vi "main_v6.vi"() -> ()   [LabVIEW 2024]
uses:
  <vilib>/Instr/_visa.llb/VISA Find Search Mode.ctl
  b10df30e-cdc0-40cb-bad4-31a4bb11d415.vi
  1b63e7fc-7b7c-41b1-b45b-52a754c22197.vi
  <vilib>/MakerHub/LINX/Public/Peripherals/Digital/Digital Write 1 Chan.vi
  <vilib>/MakerHub/LINX/Public/Peripherals/Digital/Digital Write N Chans.vi
  <vilib>/MakerHub/LINX/Private/Local IO/LinxDigitalWrite.vi
  <vilib>/MakerHub/LINX/Public/Utilities/Check Channel.vi
  <vilib>/MakerHub/LINX/Private/Local IO/Handle Errors.vi
  <vilib>/LabVIEW Open Source Project/MQTT TCP Connection/MQTT_TCP/Connection/TCPConnection.lvclass
  C:/Program Files (x86)/National Instruments/LabVIEW 2024/vi.lib/LabVIEW Open Source Project/Connection/Connection/Connection.lvclass
  <vilib>/LabVIEW Open Source Project/MQTT Client/Client class/Client.lvclass
  C:/Program Files (x86)/National Instruments/LabVIEW 2024/vi.lib/LabVIEW Open Source Project/MQTT Connection/MQTT_Base/Base Class/MQTT_Base.lvclass
  <vilib>/Instr/_visa.llb/VISA Configure Serial Port (Instr).vi
  <vilib>/MakerHub/LINX/Public/Utilities/Open Local.vi
  <vilib>/MakerHub/LINX/Private/Utilties/Generate Error.vi
  <vilib>/LabVIEW Open Source Project/MQTT Connection/MQTT_Base/Base Class/MQTT_Base.lvclass
  <vilib>/MakerHub/LINX/LMH-LINX.lvlib
panel:
  out "ambient temp":u8=6
  out "date":string
  out "is_heater_on":bool
  out "residents":u8=6
  out "activity state":i8
  out "Movement timer 2":u8
  out "door activity":bool
  out "Movement detected":bool
  out "Movement timer":u8
  out "Movement detected3":bool
  out "Is door open":bool
  out "Distance":dbl
  out "Pressure":u16
  out "Temperature":dbl
  in  "Pressure":u16
  in  "Distance":dbl
  in  "Temperature":dbl
  out "size(s)":i32
  out "unsigned byte array":u8[](array[numeric])
  out "after substring":string
  out "time string":string
  out "find list":string[](array[string])
  out "String":string
  in  "stop":bool
  in  "VISA Reciever":refnum<visa-resource-name>="ASRL1::INSTR"
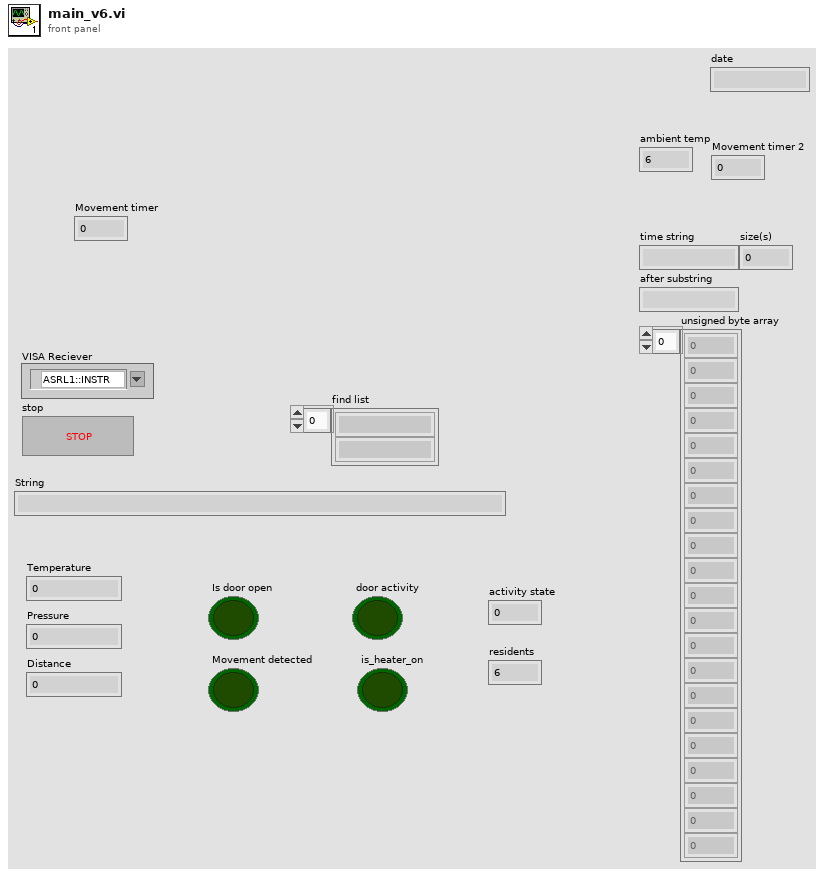
[diagram p1: front panel]
types:
  T1 = typedef "VISA Find Search Mode.ctl" = u32
  T2 = cluster{"is_door_open":bool, "is_heater_on":bool, "residents":u8, "temp":dbl, "pressure":u16, "timestamp":string, "date":string}
  T3 = typedef "LMH-LINX.lvlib/LINX Ref.ctl" = cluster{"IO":T4, "Interface":T5, "LINX Device Config":T6}
  T4 = typedef "LMH-LINX.lvlib/Platform.ctl" = enum16{"Remote", "Local"}
  T5 = typedef "LMH-LINX.lvlib/Interface.ctl" = enum16{"Serial", "TCP"}
  T6 = typedef "LMH-LINX.lvlib/Device.lvlib/LINX Device Config.ctl" = cluster{"Interface":T5, "COM Port":refnum<visa-resource-name>, "TCP Configuration":T7, "Device Family":u8, "Device ID":u8, "Device Name":string, "TCP Ref":refnum<k5>, "Channels":T8}
  T7 = typedef "LMH-LINX.lvlib/Device.lvlib/TCP Config.ctl" = cluster{"IP Address":string, "Port":u16}
  T8 = typedef "LMH-LINX.lvlib/Channels.ctl" = cluster{"DI":u8[], "DO":u8[], "AI":u8[], "AO":u8[], "PWM":u8[], "QE":u8[], "UART":u8[], "I2C 2":u8[], "SPI":u8[], "CAN":u8[], "Servo":u8[], "AI Ref (V)":dbl, "AI Resolution (Bits)":u8, "AO Ref (V)":dbl, "AO Resolution (Bits)":u8}
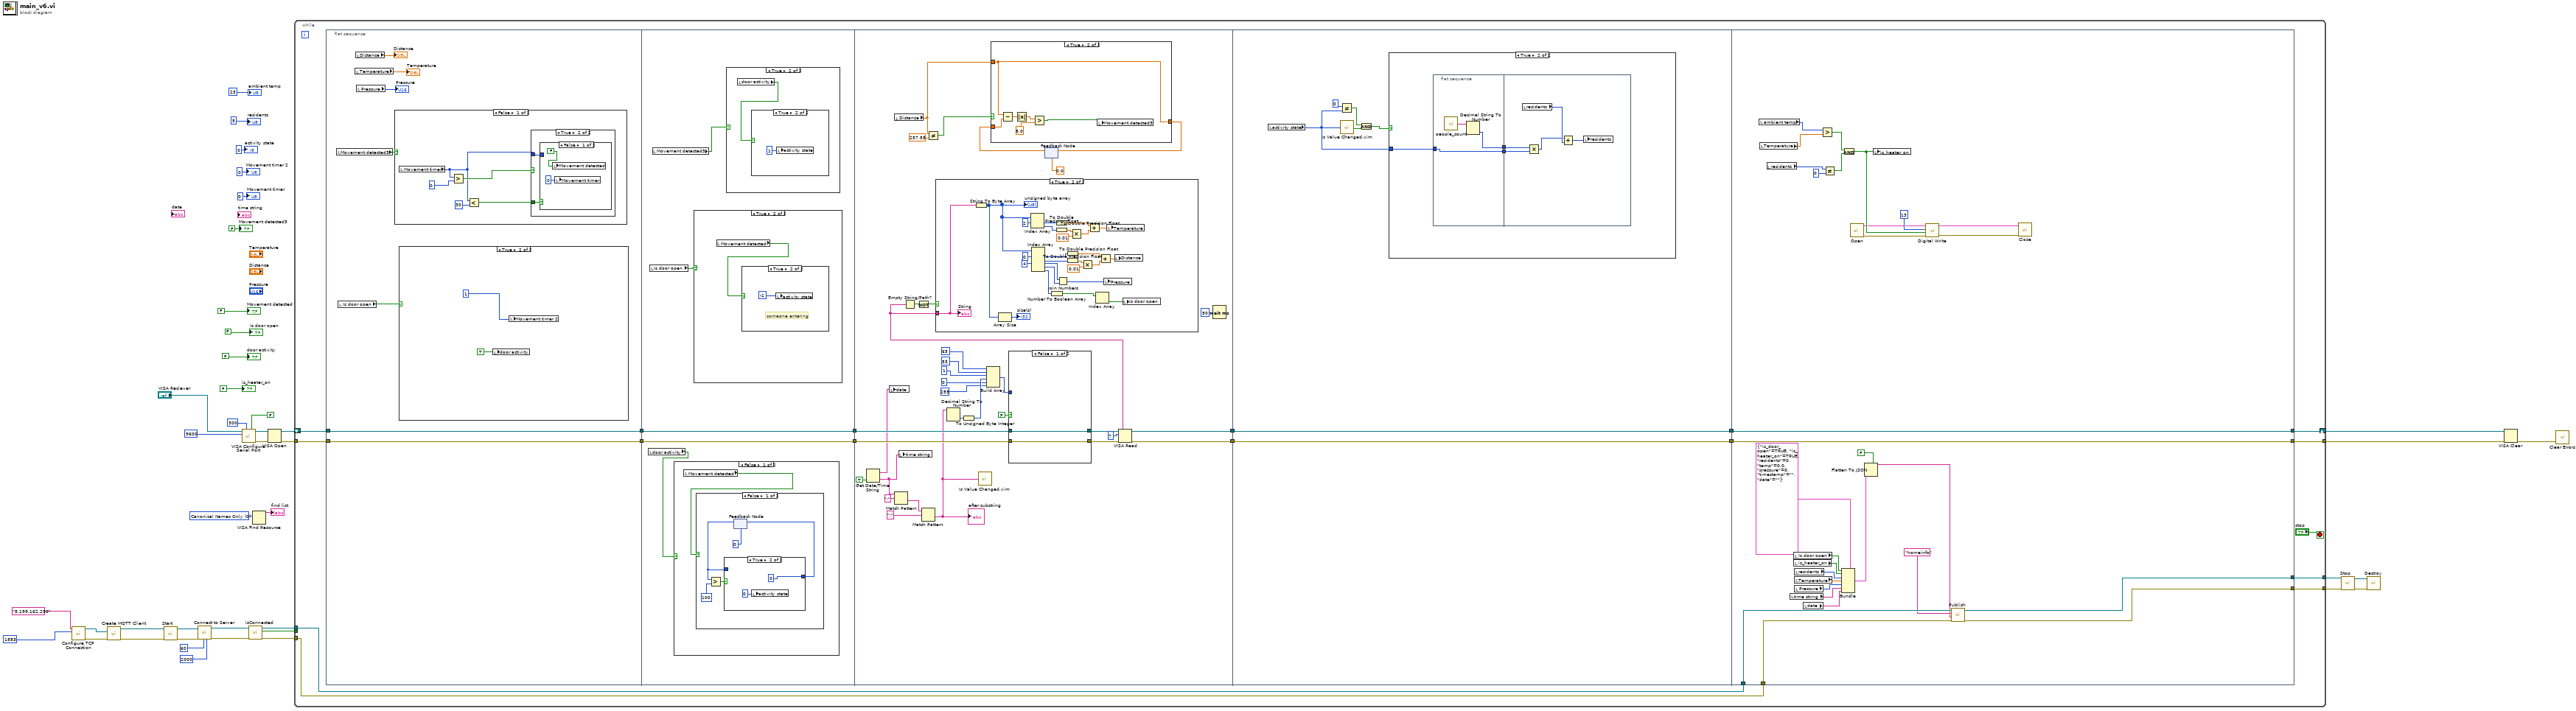
[diagram p0: block diagram]
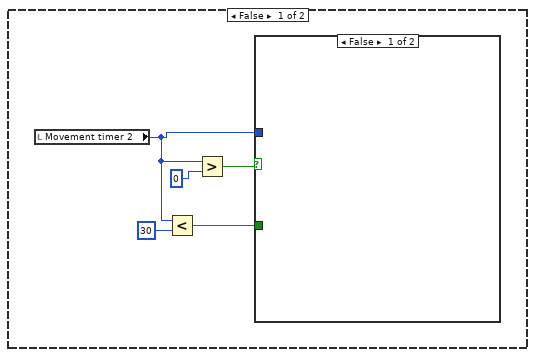
[diagram p2: hidden frame]
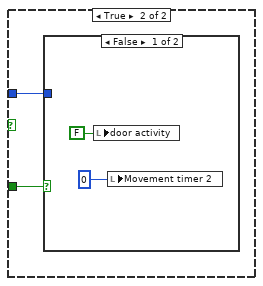
[diagram p3: hidden frame]
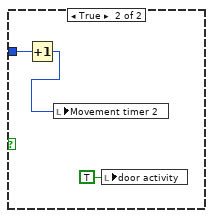
[diagram p4: hidden frame]
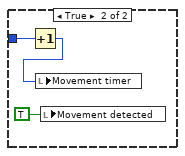
[diagram p6: hidden frame]
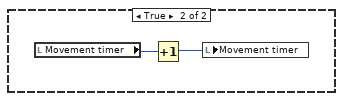
[diagram p7: hidden frame]
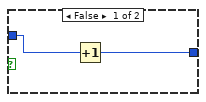
[diagram p8: hidden frame]
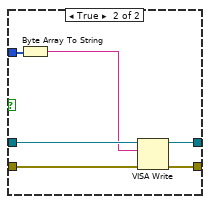
[diagram p16: hidden frame]
diagram:
  w31 = T1 0 items=["Canonical Names Only"=0, "Aliases Only"=2, "Include Matching Aliases"=3, "Include All Aliases"=4] ("Search Mode")
  n1 = call <vilib>:"Configure TCP Connection.vi"("remote port (80)"=u16 1883, "address (localhost)"="5.199.162.250") -> ("error out"=w20:errorcluster, "TCPConnection"=w19:refnum<class "TCPConnection.lvclass">)  [unwired: 8 in]
  n2 = call <vilib>:"Create MQTT Client.vi"("error in (no error)"=w20, "Connection Configuration"=w19) -> ("error out"=w13:errorcluster, "Client out"=w14:refnum<class "Client.lvclass">)  [unwired: 8 in]
  n3 = call <vilib>:"Start.vi"("error in (no error)"=w13, "MQTT_Base in"=w14) -> ("error out"=w17:errorcluster, "MQTT_Base out"=w18:refnum<class "Client.lvclass">)  [unwired: 7 in, 1 out]
  n4 = call <vilib>:"Connect to Server.vi"("timeout (2000 ms)"=2000, "Keep Alive (s)"=u16 60, "error in (no error)"=w17, "Client in"=w18) -> ("error out"=w15:errorcluster, "Client out"=w16:refnum<class "Client.lvclass">)  [unwired: 4 in, 2 out]
  n5 = call-poly "VISA Configure Serial Port"("VISA resource name"="VISA Reciever", "timeout (10sec)"=u32 300, "Enable Termination\nChar (T)"=FALSE ("Enable Termination\nChar (T)"), "baud rate (9600)"=u32 9600) -> ("VISA resource name out"=w39:refnum<visa-resource-name>, "error out"=w36:errorcluster)  [unwired: 10 in]
  n6 = call <vilib>:"isConnected.vi"("error in (no error)"=w15, "Client in"=w16) -> ("error out"=w8:errorcluster, "connected"=w7:bool, "Client out"=w9:refnum<class "Client.lvclass">)  [unwired: 7 in]
  n7 = VISA Find Resource(10:w31) -> (3:→"find list":string[])  [unwired: 2 in, 2 out]
  n8 = VISA Open(error in (no error)=w36, VISA resource name=w39) -> (VISA resource name=w38:refnum<visa-resource-name>, error out=w37:errorcluster)  [unwired: 3 in]
  n9 = while {
    shift-right: [w58] -> w34
    shift-left: w38 -> [w57]
    tunnel: w37 -> [w56]
    tunnel: [w55] -> w33
    tunnel: w9 -> [w45]
    tunnel: w8 -> [w46]
    tunnel: w7 -> [_]
    tunnel: [w44] -> w3
    tunnel: [w43] -> w2
    stop <- "stop" stop-if-true
    n10 = flat-sequence {
      tunnel: w56 -> [w65]
      tunnel: w57 -> [w66]
      tunnel: [w66] -> w54
      tunnel: [w65] -> w52
      tunnel: w54 -> [w99]
      tunnel: [w99] -> w53
      tunnel: w52 -> [w98]
      tunnel: [w98] -> w51
      tunnel: w53 -> [w141]
      tunnel: w51 -> [w140]
      tunnel: [w142] -> w50
      tunnel: [w122] -> w48
      tunnel: w50 -> [w194]
      tunnel: [w194] -> w49
      tunnel: w48 -> [w193]
      tunnel: [w193] -> w47
      tunnel: [w234] -> w55
      tunnel: [w235] -> w58
      tunnel: w49 -> [w235]
      tunnel: w47 -> [w234]
      tunnel: w46 -> [w232]
      tunnel: w45 -> [w233]
      tunnel: [w222] -> w44
      tunnel: [w221] -> w43
      frame #0 {
        n11 = local read "Movement detected3"() -> (w61:bool)
        n12 = local read "Is door open"() -> (w60:bool)
        n13 = local read "Temperature"() -> (→"Temperature":dbl)
        n14 = local read "Distance"() -> (→"Distance":dbl)
        n15 = local read "Pressure"() -> (→"Pressure":u16)
        n16 = case shown="False" w61 {
          frame False {
            n17 = local read "Movement timer"() -> (w82:u8)
            n18 = Greater?(x=w82, y=u8 0) -> (0:w83:bool)
            n19 = Less?(x=w82, y=u8 30) -> (x < y?=w81:bool)
            n20 = case shown="True" w83 {
              tunnel: w82 -> [_ w86]
              tunnel: w81 -> [_ w87]
              frame False {
              }
              frame True {
                n21 = case shown="False" w87 {
                  tunnel: w86 -> [_ w92]
                  frame False {
                    n22 = local write "Movement detected"(FALSE ("Movement detected")) -> ()
                    n23 = local write "Movement timer"(u8 0 ("Movement timer")) -> ()
                  }
                  frame True {
                    n24 = Increment(x=w92) -> (x+1=w91:u8)
                    n25 = local write "Movement timer"(w91) -> ()
                    n26 = local write "Movement detected"(TRUE ("Movement detected 2")) -> ()
                  }
                }
              }
            }
          }
          frame True {
            n27 = local read "Movement timer"() -> (w94:u8)
            n28 = Increment(x=w94) -> (x+1=w93:u8)
            n29 = local write "Movement timer"(w93) -> ()
          }
        }
        n30 = case shown="True" w60 {
          frame False {
            n31 = local read "Movement timer 2"() -> (w67:u8)
            n32 = Less?(x=w67, y=u8 30) -> (x < y?=w68:bool)
            n33 = Greater?(x=w67, y=u8 0) -> (0:w69:bool)
            n34 = case shown="False" w69 {
              tunnel: w68 -> [_ w73]
              tunnel: w67 -> [_ w72]
              frame False {
              }
              frame True {
                n35 = case shown="False" w73 {
                  tunnel: w72 -> [_ w77]
                  frame False {
                    n36 = local write "door activity"(FALSE ("door activity")) -> ()
                    n37 = local write "Movement timer 2"(u8 0 ("Movement timer 2")) -> ()
                  }
                  frame True {
                    n38 = Increment(x=w77) -> (x+1=w76:u8)
                    n39 = local write "Movement timer 2"(w76) -> ()
                    n40 = local write "door activity"(TRUE ("door activity")) -> ()
                  }
                }
              }
            }
          }
          frame True {
            n41 = local write "door activity"(TRUE ("door activity")) -> ()
            n42 = local write "Movement timer 2"(1) -> ()
          }
        }
      }
      frame #1 {
        n43 = local read "door activity"() -> (w96:bool)
        n44 = local read "Is door open"() -> (w97:bool)
        n45 = local read "Movement detected3"() -> (w95:bool)
        n46 = case shown="False" w96 {
          frame False {
            n47 = local read "Movement detected"() -> (w100:bool)
            n48 = case shown="False" w100 {
              frame False {
                n49 = feedback #1(0) -> (w102:i32)
                n50 = Greater?(x=w102, y=100) -> (0:w104:bool)
                n51 = case shown="True" w104 {
                  tunnel: w102 -> [w107 _]
                  tunnel: [w106 0] -> w101
                  frame False {
                    n52 = Increment(x=w107) -> (x+1=w106:i32)
                  }
                  frame True {
                    n53 = local write "activity state"(i8 0 ("activity state")) -> ()
                  }
                }
                n54 = feedback-in #1(w101) -> ()
              }
              frame True {
              }
            }
          }
          frame True {
          }
        }
        n55 = case shown="True" w97 {
          frame False {
          }
          frame True {
            n56 = local read "Movement detected"() -> (w112:bool)
            n57 = case shown="True" w112 {
              frame False {
              }
              frame True {
                # "someone entering"
                n58 = local write "activity state"(i8 -1 ("activity state")) -> ()
              }
            }
          }
        }
        n59 = case shown="True" w95 {
          frame False {
          }
          frame True {
            n60 = local read "door activity"() -> (w110:bool)
            n61 = case shown="True" w110 {
              frame False {
              }
              frame True {
                n62 = local write "activity state"(i8 1 ("activity state")) -> ()
              }
            }
          }
        }
      }
      frame #2 {
        n63 = Get Date/Time String(want seconds? (F)=TRUE) -> (date string=w114:string, time string=w115:string)  [unwired: 2 in]
        n64 = local write "date"(w114) -> ()
        n65 = local read "Distance"() -> (w118:dbl)
        n66 = Match Pattern(string=w115, regular expression=":") -> (after substring=w138:string)  [unwired: 1 in, 3 out]
        n67 = local write "time string"(w115) -> ()
        n68 = Match Pattern(string=w138, regular expression=":") -> (after substring=w133:string)  [unwired: 1 in, 3 out]
        "after substring" <- w133
        n69 = Not Equal?(x=w118, y=257.55) -> (x != y?=w119:bool)
        n70 = Decimal String To Number(string=w133) -> (number=w131:i32)  [unwired: 2 in, 1 out]
        n71 = To Unsigned Byte Integer(number=w131) -> (unsigned 8bit integer=w128:u8)
        n72 = call "Is Value Changed.vim"("value"=w133) -> ()  [unwired: 1 out]
        n73 = Build Array(u8 65 ("element"), u8 53 ("element"), u8 1 ("element"), w128, u8 0 ("element"), u8 255 ("element")) -> (w132:u8[])
        n74 = case shown="False" FALSE {
          tunnel: [w155 w161] -> w143
          tunnel: w141 -> [w155 w160]
          tunnel: w140 -> [w154 w159]
          tunnel: w132 -> [_ w158]
          tunnel: [w154 w156] -> w123
          frame False {
          }
          frame True {
            n75 = Byte Array To String(unsigned byte array=w158) -> (string=w157:string)
            n76 = VISA Write(VISA resource name=w160, write buffer=w157, error in (no error)=w159) -> (VISA resource name out=w161:refnum<visa-resource-name>, error out=w156:errorcluster)  [unwired: 1 out]
          }
        }
        n77 = feedback #2(0.0) -> (w117:dbl)
        n78 = case shown="True" w119 {
          tunnel: w118 -> [_ w153]
          tunnel: [w147 w153] -> w116
          tunnel: w117 -> [w147 w152]
          frame False {
          }
          frame True {
            n79 = Subtract(x=w153, y=w152) -> (x-y=w151:dbl)
            n80 = Absolute Value(x=w151) -> (abs(x)=w150:dbl)
            n81 = Greater?(x=w150, y=8.0) -> (0:w148:bool)
            n82 = local write "Movement detected3"(w148) -> ()
          }
        }
        n83 = feedback-in #2(w116) -> ()
        n84 = VISA Read(VISA resource name=w143, byte count=u32 7, error in (no error)=w123) -> (VISA resource name out=w142:refnum<visa-resource-name>, read buffer=w139:string, error out=w122:errorcluster)  [unwired: 1 out]
        n85 = Empty String/Path?(string/path=w139) -> (empty?=w146:bool)
        n86 = Not(x=w146) -> (.not. x?=w145:bool)
        n87 = case shown="True" w145 {
          tunnel: w139 -> [_ w187]
          frame False {
          }
          frame True {
            n88 = String To Byte Array(string=w187) -> (unsigned byte array=w177:u8[])
            "unsigned byte array" <- w177
            n89 = Array Size(array=w177) -> (size(s)=→"size(s)":i32)
            n90 = Index Array(array=w177, index #1=2 ("index")) -> (element #1=w185:u8, element #2=w184:u8)  [unwired: 1 in]
            n91 = Index Array(array=w177, index #1=0 ("index"), index #3=4 ("index")) -> (element #1=w171:u8, element #2=w170:u8, element #3=w168:u8, element #4=w167:u8, element #5=w164:u8)  [unwired: 3 in]
            n92 = Number To Boolean Array(number=w164) -> (Boolean array=w163:bool[])
            n93 = To Double Precision Float(number=w185) -> (double precision float=w180:dbl)
            n94 = To Double Precision Float(number=w184) -> (double precision float=w183:dbl)
            n95 = Join Numbers(hi=w168, lo=w167) -> ((hi.lo)=w166:u16)
            n96 = To Double Precision Float(number=w171) -> (double precision float=w172:dbl)
            n97 = To Double Precision Float(number=w170) -> (double precision float=w175:dbl)
            n98 = Multiply(x=w183, y=0.01) -> (x*y=w181:dbl)
            n99 = Multiply(x=w175, y=0.01) -> (x*y=w173:dbl)
            n100 = Add(x=w180, y=w181) -> (x+y=w179:dbl)
            n101 = Index Array(array=w163) -> (element=w162:bool)  [unwired: 1 in]
            n102 = Add(x=w172, y=w173) -> (x+y=w169:dbl)
            n103 = local write "Pressure"(w166) -> ()
            n104 = local write "Temperature"(w179) -> ()
            n105 = local write "Distance"(w169) -> ()
            n106 = local write "Is door open"(w162) -> ()
            "String" <- w187
          }
        }
        n107 = Wait (ms)(milliseconds to wait=u32 50) -> ()  [unwired: 1 out]
      }
      frame #3 {
        n108 = local read "activity state"() -> (w192:i8)
        n109 = Not Equal?(x=i8 0, y=w192) -> (x != y?=w190:bool)
        n110 = call "Is Value Changed.vim"("value"=w192) -> ("changed or first call?"=w189:bool)
        n111 = And(x=w190, y=w189) -> (x .and. y?=w188:bool)
        n112 = case shown="True" w188 {
          tunnel: w192 -> [_ w197]
          frame False {
          }
          frame True {
            n113 = flat-sequence {
              tunnel: w197 -> [w199]
              tunnel: [w199] -> w196
              tunnel: [w198] -> w195
              tunnel: w196 -> [w202]
              tunnel: w195 -> [w201]
              frame #0 {
                n114 = call "people_count.vi"() -> ("data out"=w200:string)  [unwired: 1 in]
                n115 = Decimal String To Number(string=w200) -> (number=w198:i32)  [unwired: 2 in, 1 out]
              }
              frame #1 {
                n116 = local read "residents"() -> (w204:u8)
                n117 = Multiply(x=w201, y=w202) -> (x*y=w203:i32)
                n118 = Add(x=w203, y=w204) -> (x+y=w205:i32)
                n119 = local write "residents"(w205) -> ()
              }
            }
          }
        }
      }
      frame #4 {
        n120 = local read "ambient temp"() -> (w217:u8)
        n121 = local read "Temperature"() -> (w216:dbl)
        n122 = local read "residents"() -> (w215:u8)
        n123 = local read "time string"() -> (w220:string)
        n124 = local read "Is door open"() -> (w224:bool)
        n125 = local read "is_heater_on"() -> (w223:bool)
        n126 = local read "residents"() -> (w225:u8)
        n127 = local read "Temperature"() -> (w226:dbl)
        n128 = local read "Pressure"() -> (w227:u16)
        n129 = local read "date"() -> (w219:string)
        n130 = Greater?(x=w217, y=w216) -> (0:w213:bool)
        n131 = Not Equal?(x=w215, y=u8 0) -> (x != y?=w212:bool)
        n132 = Bundle(cluster=T2 {"is_door_open"=TRUE, "is_heater_on"=TRUE, "residents"=0, "temp"=0.0, "pressure"=0, "timestamp"="", "date"=""} ("anything"), "is_door_open"=w224, "is_heater_on"=w223, "residents"=w225, "temp"=w226, "pressure"=w227, "timestamp"=w220, "date"=w219) -> (w229:T2)
        n133 = And(x=w213, y=w212) -> (x .and. y?=w211:bool)
        n134 = call-poly <vilib>:"Open.vi"() -> ("Error Out"=w208:errorcluster, "LINX Resource"=w209:T3)  [unwired: 9 in, 1 out]
        n135 = Flatten To JSON(enable LabVIEW extensions? (T)=FALSE, anything=w229) -> (JSON string=w228:string)  [unwired: 1 in, 1 out]
        n136 = local write "is_heater_on"(w211) -> ()
        n137 = call-poly <vilib>:"Digital Write.vi"("Error In"=w208, "Output Value"=w211, "DO Channel"=u8 13, "LINX Resource"=w209) -> ("Error Out"=w206:errorcluster, "LINX Resource"=w207:T3)  [unwired: 6 in]
        n138 = call <vilib>:"Publish.vi"("error in (no error)"=w232, "Payload"=w228, "Topic Name (empty: Payload name)"="homeinfo", "Client in"=w233) -> ("error out"=w221:errorcluster, "Client out"=w222:refnum<class "Client.lvclass">)  [unwired: 5 in, 1 out]
        n139 = call <vilib>:"Close.vi"("Error In"=w206, "LINX Resource"=w207) -> ()  [unwired: 9 in, 1 out]
      }
    }
  }
  n140 = call <vilib>:"Stop.vi"("error in (no error)"=w2, "MQTT_Base in"=w3) -> ("error out"=w4:errorcluster, "MQTT_Base out"=w5:refnum<class "Client.lvclass">)  [unwired: 7 in, 1 out]
  n141 = call <vilib>:"Destroy.vi"("error in (no error)"=w4, "MQTT_Base in"=w5) -> ()  [unwired: 8 in, 2 out]
  n142 = VISA Clear(VISA resource name=w34, error in (no error)=w33) -> (error out=w35:errorcluster)  [unwired: 1 out]
  n143 = call <vilib>:"Clear Errors.vi"("error in (no error)"=w35) -> ()  [unwired: 5 in, 2 out]
  "Movement detected3" <- FALSE ("Movement detected")
  "Movement timer" <- u8 0 ("Movement timer")
  "Movement detected" <- FALSE ("Movement detected")
  "Is door open" <- FALSE ("Is door open")
  "door activity" <- FALSE ("Is door open")
  "Movement timer 2" <- u8 0 ("Movement timer")
  "activity state" <- i8 0 ("activity state")
  "residents" <- u8 5
  "is_heater_on" <- FALSE ("Is door open")
  "ambient temp" <- u8 23
